vi "Parse Results (table).vi"(8 "error in (no error)":errorcluster, 9 "Input Gain":T1=[{"Channel"="AI1", "Gain"=1.0}, {"Channel"="AI2", "Gain"=1.0}, {"Channel"="AI3", "Gain"=1.0}, {"Channel"="AI4", "Gain"=1.0}, {"Channel"="AI5", "Gain"=1.0}, {"Channel"="AI6", "Gain"=1.0}, {"Channel"="AI7", "Gain"=1.0}, {"Channel"="AI8", "Gain"=1.0}, {"Channel"="AI9", "Gain"=1.0}, {"Channel"="AI10", "Gain"=1.0}, {"Channel"="AI11", "Gain"=1.0}, {"Channel"="AI12", "Gain"=1.0}, {"Channel"="AI13", "Gain"=1.0}, {"Channel"="AI14", "Gain"=1.0}, {"Channel"="AI15", "Gain"=1.0}, {"Channel"="AI16", "Gain"=1.0}], 10 "DAQ Config":T3 {"AO terminal config" items=[""=-1, "differential"=10106, "pseudodifferential"=12529]; "AI terminal config" items=[""=-1, "differential"=10106, "pseudodifferential"=12529]; "AI.Coupling" items=[""=0, "AC"=10045, "DC"=10050, "GND"=10066]}, 11 "Results (Dictionary)":cluster{"key":string, "value":dbl}[](array[cluster])) -> (0 "error out":errorcluster, 2 "Table":string[][](table), 3 "Results (Dictionary) out":cluster{"key":string, "value":dbl}[](array[cluster]))   [LabVIEW 2019, in "Instrument.Lockin.lvlib" / "Instrument UI.Lockin.lvclass"]
uses:
  Instrument UI.Lockin.lvclass
  Instrument.DAQ/Typedefs/DAQ.Configuration--Cluster--Array.ctl
  Instrument.DAQ/Typedefs/DAQ.Configuration--Cluster.ctl
  Instrument.DAQ/Typedefs/DAQ.Config.AO.Range--enum.ctl
  Instrument.DAQ/Typedefs/DAQ.Config.AI.Range--enum.ctl
  Instrument.DAQ/Typedefs/DAQ.Config.AI.Coupling--enum.ctl
  Instrument.DAQ/Typedefs/DAQ.TerminalConfiguration--ring.ctl
  Instrument.DAQ/Typedefs/Channel.Gain--Cluster--Array.ctl
  Instrument.DAQ/Typedefs/Channel.Gain--Cluster.ctl
  Instrument.Lockin/Typedefs/Results Type--Enum.ctl
  Instrument.Lockin/Instrument.Lockin.lvclass
  Instrument.DAQ/Instrument.DAQ.lvclass
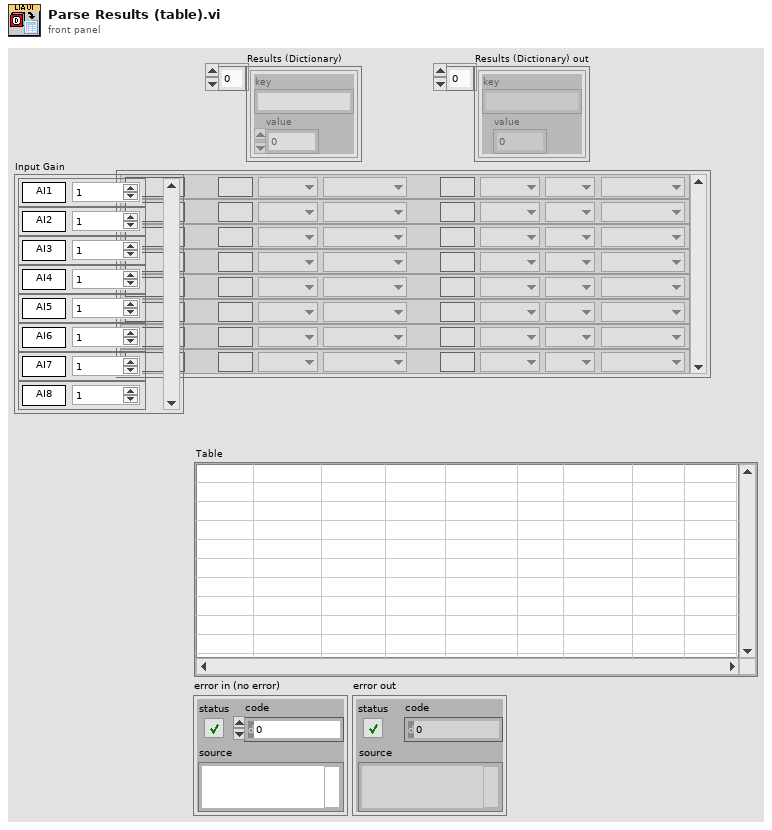
[diagram p1: front panel]
types:
  T1 = typedef "Instrument.Lockin.lvlib/Instrument.DAQ.lvclass/Channel.Gain--Cluster--Array.ctl" = T2[]
  T2 = typedef "Instrument.Lockin.lvlib/Instrument.DAQ.lvclass/Channel.Gain--Cluster.ctl" = cluster{"Channel":string, "Gain":dbl}
  T3 = typedef "Instrument.Lockin.lvlib/Instrument.DAQ.lvclass/DAQ.Configuration--Cluster--Array.ctl" = T4[]
  T4 = typedef "Instrument.Lockin.lvlib/Instrument.DAQ.lvclass/DAQ.Configuration--Cluster.ctl" = cluster{"Device":string, "AO.Ch":string, "AO.Range":T5, "AI.Ch":string, "AI.Range":T6, "AI.Coupling":T7, "AI terminal config":T8, "AO terminal config":T8}
  T5 = typedef "Instrument.Lockin.lvlib/Instrument.DAQ.lvclass/DAQ.Config.AO.Range--enum.ctl" = enum16{"±0.1", "±1.0", "±10.0", ""}
  T6 = typedef "Instrument.Lockin.lvlib/Instrument.DAQ.lvclass/DAQ.Config.AI.Range--enum.ctl" = enum16{"±0.316", "±1.00", "±3.16", "±10.0", "±31.6", "±42.4", ""}
  T7 = typedef "Instrument.Lockin.lvlib/Instrument.DAQ.lvclass/DAQ.Config.AI.Coupling--enum.ctl" = u16
  T8 = typedef "Instrument.Lockin.lvlib/Instrument.DAQ.lvclass/DAQ.TerminalConfiguration--ring.ctl" = i32
  T9 = typedef "Instrument.Lockin.lvlib/Instrument.Lockin.lvclass/Results Type--Enum.ctl" = enum16{"X", "Y", "R", "Theta", "Mean"}
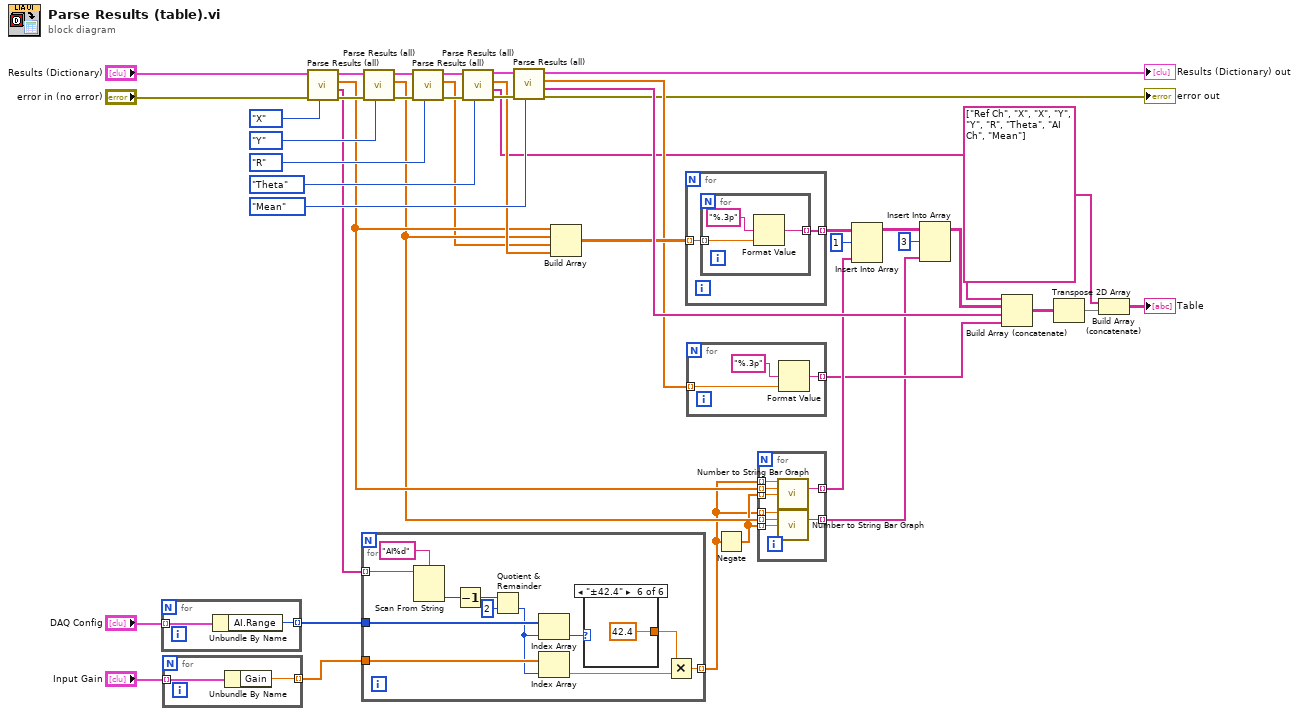
[diagram p0: block diagram]
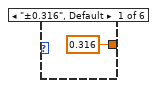
[diagram p2: hidden frame]
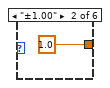
[diagram p3: hidden frame]
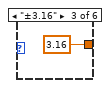
[diagram p4: hidden frame]
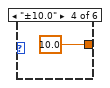
[diagram p5: hidden frame]
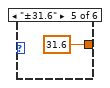
[diagram p6: hidden frame]
diagram:
  n1 = for {
    tunnel: "DAQ Config" -> [w46] mode=indexing
    tunnel: [w45] -> w6 mode=indexing
    n2 = Unbundle By Name(w46) -> ("AI.Range"=w45:T6)
  }
  n3 = for {
    tunnel: "Input Gain" -> [w48] mode=indexing
    tunnel: [w47] -> w1 mode=indexing
    n4 = Unbundle By Name(w48) -> ("Gain"=w47:dbl)
  }
  n5 = call "Parse Results (all).vi"("Type"=Results_Type--Enum."X", "error in (no error)"="error in (no error)", "Results (Dictionary)"="Results (Dictionary)") -> ("error out"=w44:errorcluster, "Names"=w12:string[], "Data"=w20:dbl[], "Results (Dictionary)"=w43:cluster{"key":string, "value":dbl}[])  [unwired: 5 in]
  n6 = for {
    tunnel: w12 -> [w60] mode=indexing
    tunnel: w6 -> [w55]
    tunnel: w1 -> [w54]
    tunnel: [w50] -> w3 mode=indexing
    n7 = Scan From String(format string="AI%d", input string=w60) -> (output 1=w58:i32)  [unwired: 3 in, 3 out]
    n8 = Decrement(x=w58) -> (x-1=w57:i32)
    n9 = Quotient & Remainder(x=w57, y=2) -> (floor(x/y)=w49:i32)  [unwired: 1 out]
    n10 = Index Array(array=w55, index=w49) -> (element=w53:T6)
    n11 = Index Array(array=w54, index=w49) -> (element=w51:dbl)
    n12 = case shown="\"±42.4\"" w53 {
      tunnel: [0.316 1.0 3.16 10.0 31.6 42.4] -> w52
      frame "±0.316", Default {
      }
      frame "±1.00" {
      }
      frame "±3.16" {
      }
      frame "±10.0" {
      }
      frame "±31.6" {
      }
      frame "±42.4" {
      }
    }
    n13 = Multiply(x=w52, y=w51) -> (x*y=w50:dbl)
  }
  n14 = call "Parse Results (all).vi"("Type"=Results_Type--Enum."Y", "error in (no error)"=w44, "Results (Dictionary)"=w43) -> ("error out"=w42:errorcluster, "Data"=w19:dbl[], "Results (Dictionary)"=w41:cluster{"key":string, "value":dbl}[])  [unwired: 5 in, 1 out]
  n15 = call "Parse Results (all).vi"("Type"=Results_Type--Enum."R", "error in (no error)"=w42, "Results (Dictionary)"=w41) -> ("error out"=w37:errorcluster, "Data"=w18:dbl[], "Results (Dictionary)"=w38:cluster{"key":string, "value":dbl}[])  [unwired: 5 in, 1 out]
  n16 = call "Parse Results (all).vi"("Type"=Results_Type--Enum."Theta", "error in (no error)"=w37, "Results (Dictionary)"=w38) -> ("error out"=w40:errorcluster, "Names"=w9:string[], "Data"=w22:dbl[], "Results (Dictionary)"=w39:cluster{"key":string, "value":dbl}[])  [unwired: 5 in]
  n17 = call "Parse Results (all).vi"("Type"=Results_Type--Enum."Mean", "error in (no error)"=w40, "Results (Dictionary)"=w39) -> ("error out"=→"error out":errorcluster, "Names"=w31:string[], "Data"=w25:dbl[], "Results (Dictionary)"=→"Results (Dictionary) out":cluster{"key":string, "value":dbl}[])  [unwired: 5 in]
  n18 = Build Array(w20, w19, w18, w22) -> (w26:dbl[][])
  n19 = for {
    tunnel: [w67] -> w17 mode=indexing
    tunnel: w26 -> [w68] mode=indexing
    n20 = for {
      tunnel: [w71] -> w67 mode=indexing
      tunnel: w68 -> [w70] mode=indexing
      n21 = Format Value(format string="%.3p", value (0)=w70) -> (output string=w71:string)  [unwired: 1 in]
    }
  }
  n22 = for {
    tunnel: w25 -> [w73] mode=indexing
    tunnel: [w72] -> w8 mode=indexing
    n23 = Format Value(format string="%.3p", value (0)=w73) -> (output string=w72:string)  [unwired: 1 in]
  }
  n24 = Negate(x=w3) -> (-x=w11:dbl[])
  n25 = for {
    tunnel: w11 -> [w82] mode=indexing
    tunnel: w3 -> [w81] mode=indexing
    tunnel: w11 -> [w80] mode=indexing
    tunnel: w3 -> [w79] mode=indexing
    tunnel: w20 -> [w78] mode=indexing
    tunnel: w19 -> [w77] mode=indexing
    tunnel: [w76] -> w7 mode=indexing
    tunnel: [w75] -> w14 mode=indexing
    n26 = call "Number to String Bar Graph.vi"("Scale Max"=w79, "Numeric"=w78, "Scale Min"=w80) -> ("element"=w75:string)  [unwired: 12 in]
    n27 = call "Number to String Bar Graph.vi"("Scale Max"=w81, "Numeric"=w77, "Scale Min"=w82) -> ("element"=w76:string)  [unwired: 12 in]
  }
  n28 = Insert Into Array(array=w17, index (row)=1, new element=w14) -> (w15:string[][])  [unwired: 1 in]
  n29 = Insert Into Array(array=w15, index (row)=3, new element=w7) -> (w10:string[][])  [unwired: 1 in]
  n30 = Build Array (concatenate)(w9, w10, w31, w8) -> (w30:string[][])
  n31 = Transpose 2D Array(2D array=w30) -> (transposed array=w29:string[][])
  n32 = Build Array (concatenate)(string[] ["Ref Ch", "X", "X", "Y", "Y", "R", "Theta", "AI Ch", "Mean"] ("Names"), w29) -> (→"Table":string[][])
